vi "Change_target_filename.vi"(4 "App Name":string="My Application", 6 "New Version":string, 7 "index":i32, 8 "error in (no error)":errorcluster, 11 "Builder in":refnum<class "Builder.lvclass">) -> (0 "error out":errorcluster, 3 "Builder out":refnum<class "Builder.lvclass">)   [LabVIEW 2021, in "App-Builder Library.lvlib" / "Builder.lvclass"]
uses:
  Builder.lvclass
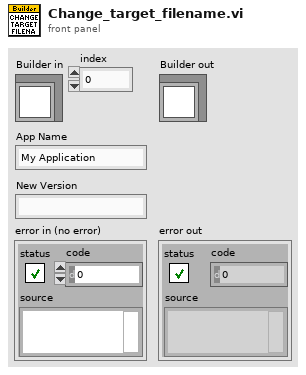
[diagram p1: front panel]
types:
  T1 = typedef "App-Builder Library.lvlib/Builder.lvclass/Build object type.ctl" = enum16{"EXE", "RT EXE", "Deployable Packed"}
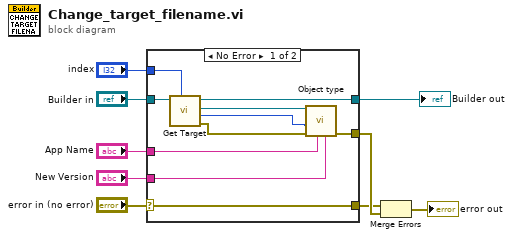
[diagram p0: block diagram]
diagram:
  n1 = case shown="No Error" "error in (no error)" {
    selector: "error in (no error)" -> [w12 w20]
    tunnel: "Builder in" -> [w19 w21]
    tunnel: "index" -> [w18 _]
    tunnel: [w17 w21] -> w7
    tunnel: "App Name" -> [w16 _]
    tunnel: "New Version" -> [w14 _]
    tunnel: [w13 _] -> w4
    tunnel: [w12 w20] -> w1
    frame No Error {
      n2 = call "Get Target.vi"("index"=w18, "Builder in"=w19) -> ("error out"=w10:errorcluster, "Build Object type"=w15:T1, "element"=w11:refnum<vi>, "Builder out"=w17:refnum<class "Builder.lvclass">)  [unwired: 6 in]
      n3 = call "Object type.vi"("New version"=w14, "App Name"=w16, "error in"=w10, "Build Object type"=w15, "Project Item Ref"=w11) -> ("error out"=w13:errorcluster)  [unwired: 6 in]
    }
    frame Error {
    }
  }
  "Builder out" <- w7
  n4 = Merge Errors(w1, w4) -> (→"error out":errorcluster)
